vi "Read PCC DeviceID.vi"(8 "error in":errorcluster, 11 "Startup Optimization in":refnum<class "Startup Optimization.lvclass">) -> (0 "error out":errorcluster, 2 "DeviceID":T1, 3 "dup Startup Optimization":refnum<class "Startup Optimization.lvclass">)   [LabVIEW 2018, in "Startup Optimization Actor.lvlib" / "Startup Optimization.lvclass"]
uses:
  Startup Optimization.lvclass
  <vilib>/ORNL/CSEISMIC DDS/CSEISMIC DDS Base/Data Types/Controls/DeviceID.ctl
  Startup Optimization.lvclass/Startup Optimization.ctl
  <vilib>/ORNL/CSEISMIC DDS/CSEISMIC DDS Base/CSEISMIC DDS.lvclass
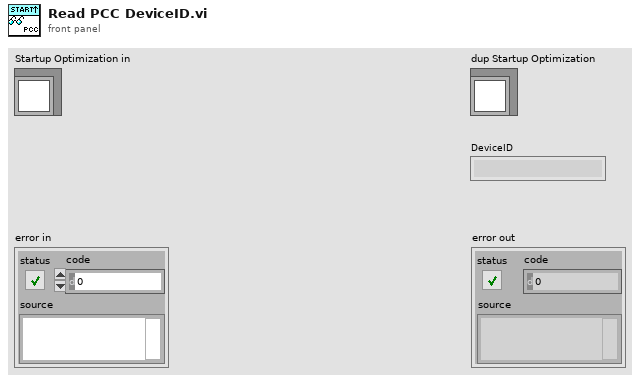
[diagram p1: front panel]
types:
  T1 = typedef "CSEISMIC DDS.lvlib/CSEISMIC DDS.lvclass/DeviceID.ctl" = string
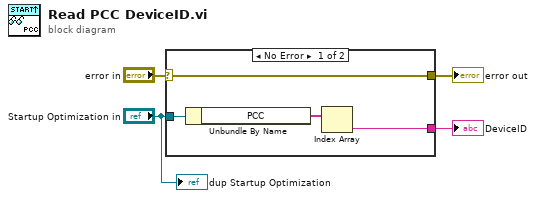
[diagram p0: block diagram]
diagram:
  n1 = case shown="No Error" "error in" {
    selector: "error in" -> [w5 w9]
    tunnel: "Startup Optimization in" -> [w8 _]
    tunnel: [w7 _] -> w4
    tunnel: [w5 w9] -> w2
    frame No Error {
      n2 = Unbundle By Name(w8) -> ("PCC"=w6:T1[])
      n3 = Index Array(array=w6) -> (element=w7:T1)  [unwired: 1 in]
    }
    frame Error {
    }
  }
  "DeviceID" <- w4
  "error out" <- w2
  "dup Startup Optimization" <- "Startup Optimization in"
